vi "Get Active Plugins.vi"(8 "error in (no error)":errorcluster) -> (0 "error out":errorcluster, 2 "Plugins":string[](array[string]))   [LabVIEW 2020, in "UI Configuration Manager.lvclass"]
uses:
  UI Configuration Manager.lvclass
  Framework/Configuration Manager/Configuration Manager.lvclass
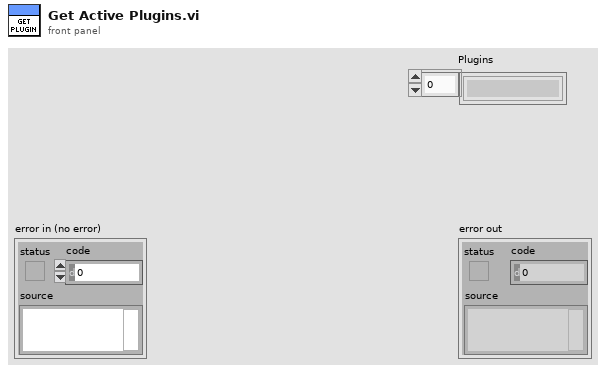
[diagram p1: front panel]
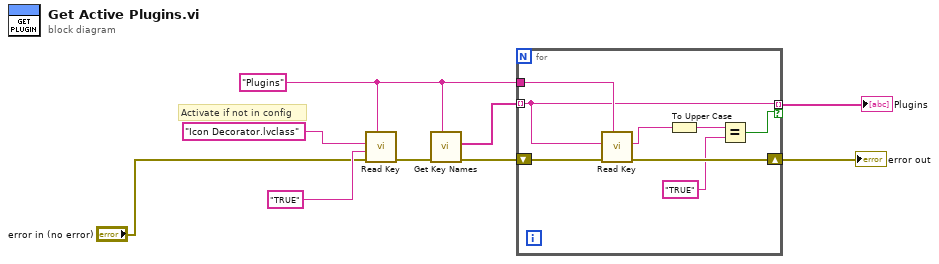
[diagram p0: block diagram]
diagram:
  w1 = "Plugins" ("section")
  # "Activate if not in config"
  n1 = call "Read Key.vi"("section"=w1, "error in (no error)"="error in (no error)", "default value"="TRUE", "key"="Icon Decorator.lvclass") -> ("error out"=w3:errorcluster)  [unwired: 6 in, 1 out]
  n2 = call "Get Key Names.vi"("Section"=w1, "error in (no error)"=w3) -> ("error out"=w2:errorcluster, "Keys"=w4:string[])  [unwired: 8 in]
  n3 = for {
    shift-right: [w16] -> w9
    shift-left: w2 -> [w17]
    tunnel: w4 -> [w14] mode=indexing
    tunnel: w1 -> [w15]
    tunnel: [w14] -> w8 mode=indexing if=w10
    n4 = call "Read Key.vi"("section"=w15, "error in (no error)"=w17, "key"=w14) -> ("error out"=w16:errorcluster, "value"=w13:string)  [unwired: 7 in]
    n5 = To Upper Case(1:w13) -> (0:w12:string)
    n6 = Equal?(x=w12, y="TRUE") -> (x = y?=w10:bool)
  }
  "error out" <- w9
  "Plugins" <- w8
